vi "Write Boolean.vi"(7 "key":string, 8 "error in (no error)":errorcluster, 9 "Value":bool, 11 "Configuration File In":refnum<class "Configuration File.lvclass">) -> (0 "error out":errorcluster, 3 "Configuration File Out":refnum<class "Configuration File.lvclass">)   [LabVIEW 2020, in "Configuration File.lvclass"]
doc: "High-level function for writing configuration file data from process class."
uses:
  Configuration File.lvclass
  Base/Base.lvclass/Base.ctl
  Base/Public/Read Base Name.vi
  Process/Public/Read Name.vi
  <vilib>/Utility/config.llb/Write Key (Boolean).vi
  Process/Process.lvclass
  Base/Base.lvclass
  <vilib>/Utility/config.llb/NI_LVConfig.lvlib
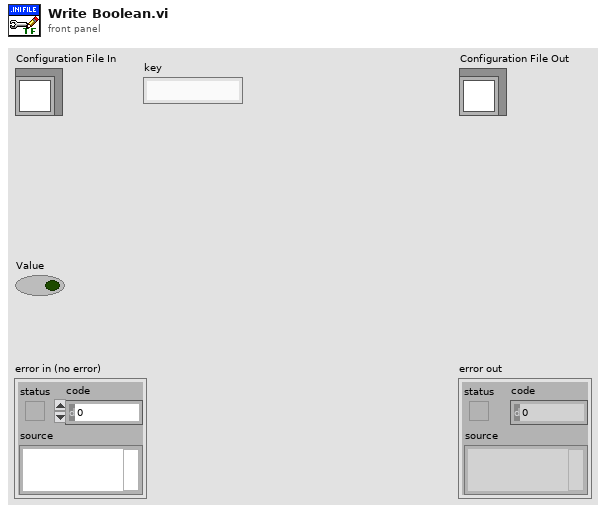
[diagram p1: front panel]
types:
  T1 = typedef "NI_LVConfig.lvlib/Config Data RefNum.ctl" = refnum<k1>
  T2 = typedef "Semaphore RefNum" = refnum<k1>
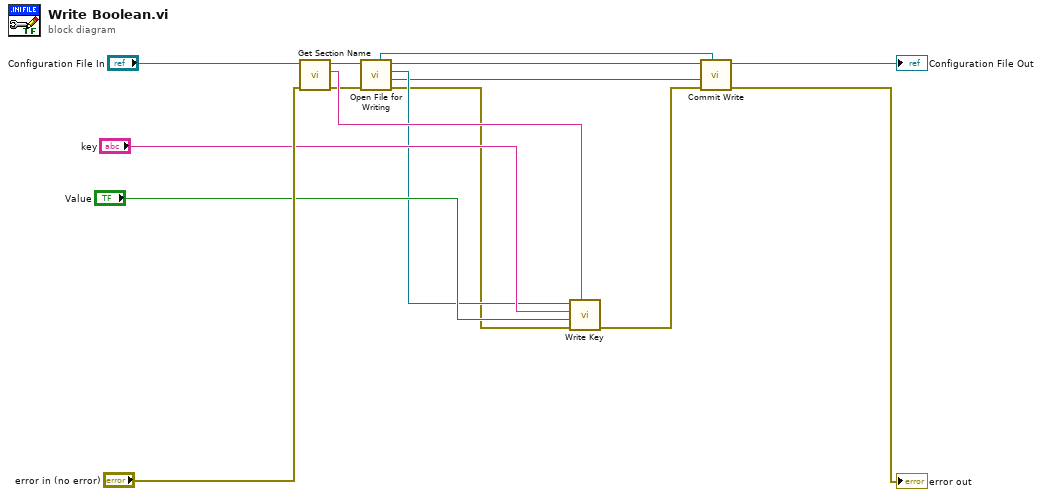
[diagram p0: block diagram]
diagram:
  n1 = call "Get Section Name.vi"("error in (no error)"="error in (no error)", "Configuration File In"="Configuration File In") -> ("error out"=w8:errorcluster, "Section Name"=w11:string, "Configuration File Out"=w6:refnum<class "Configuration File.lvclass">)  [unwired: 7 in]
  n2 = call "Open File for Writing.vi"("error in (no error)"=w8, "Configuration File in"=w6) -> ("error out"=w7:errorcluster, "File was Open?"=w2:bool, "refnum out"=w9:T1, "Configuration File out"=w5:refnum<class "Configuration File.lvclass">, "semaphore"=w1:T2)  [unwired: 5 in]
  n3 = call-poly <vilib>:"Write Key.vi"("section"=w11, "error in (no error)"=w7, "value"="Value", "key"="key", "refnum"=w9) -> ("error out"=w4:errorcluster)  [unwired: 4 in, 2 out]
  n4 = call "Commit Write.vi"("Semaphore"=w1, "error in (no error)"=w4, "Leave File Open?"=w2, "Configuration File In"=w5) -> ("error out"=→"error out":errorcluster, "Configuration File Out"=→"Configuration File Out":refnum<class "Configuration File.lvclass">)  [unwired: 6 in]
